vi "Pot HDI.vi"(8 "error in (no error)":errorcluster, 11 "SyringeTool Class in":refnum<class "SyringeTool Class.lvclass">) -> (0 "error out":errorcluster, 3 "SyringeTool Class out":refnum<class "SyringeTool Class.lvclass">)   [LabVIEW 2011, in "SyringeTool Class.lvclass"]
uses:
  SyringeTool Class.lvclass
  WorkTable Class/WorkTable Class.lvclass
  Vec3d Class/Vec3d Class.lvclass
panel:
  in  "Slot":u32
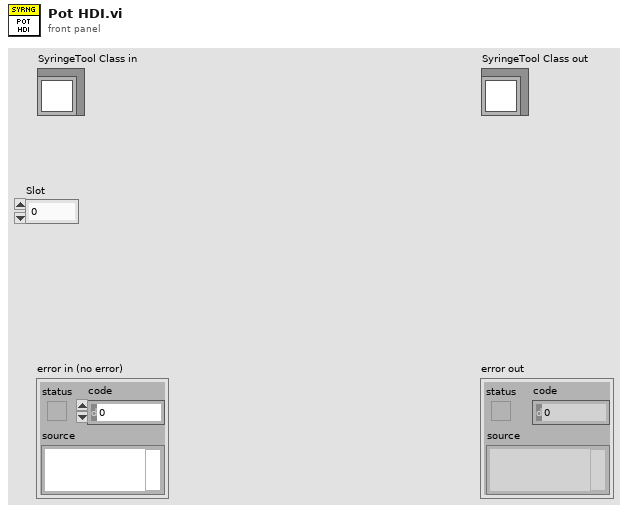
[diagram p1: front panel]
types:
  T1 = typedef "Worktable_HDI Slot.ctl" = cluster{"HDI Assembly State":enum16{"Empty", "Populated"}, "HDI Type":enum16{"HDI", "Polyimide"}, "Vacuum Channel":u32, "Location/Orientation":T2}
  T2 = typedef "Position_Orientation.ctl" = cluster{"Center":refnum<class "Vec3d Class.lvclass">, "Orientation":refnum<class "Orient3d Class.lvclass">}
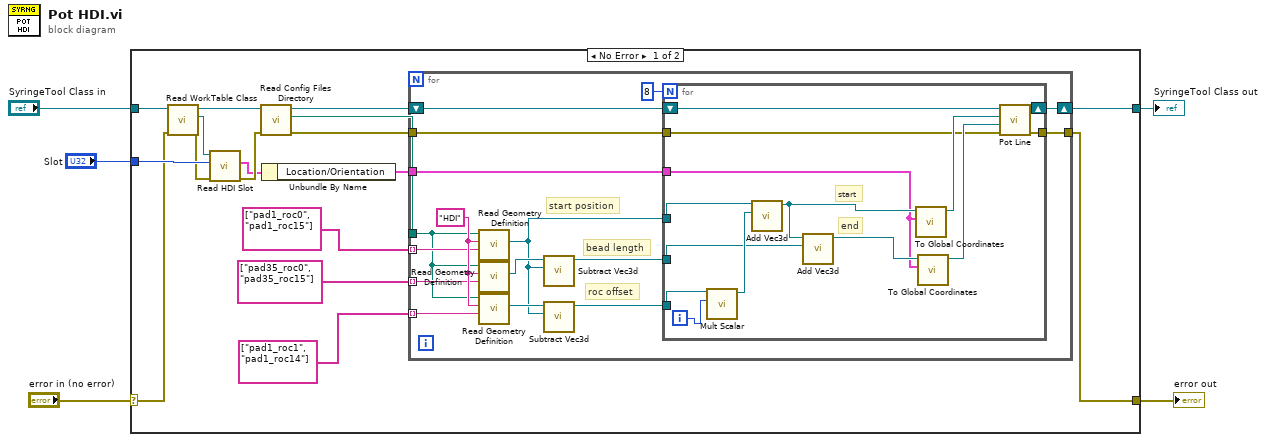
[diagram p0: block diagram]
diagram:
  n1 = case shown="No Error" "error in (no error)" {
    selector: "error in (no error)" -> [w8 w54]
    tunnel: [w6 w54] -> w4
    tunnel: [w14 w53] -> w2
    tunnel: "SyringeTool Class in" -> [w22 w53]
    tunnel: "Slot" -> [w20 _]
    frame No Error {
      n2 = call-dynamic "Read WorkTable Class.vi"("error in"=w8, "Gantry Class in"=w22) -> ("error out"=w19:errorcluster, "WorkTable Class.lvclass"=w21:refnum<class "WorkTable Class.lvclass">, "Gantry Class out"=w18:refnum<class "SyringeTool Class.lvclass">)  [unwired: 7 in]
      n3 = call-dynamic "Read HDI Slot.vi"("error in"=w19, "HDI Slot Number"=w20, "WorkTable in"=w21) -> ("error out"=w17:errorcluster, "HDI Slot"=w16:T1)  [unwired: 6 in, 1 out]
      n4 = call-dynamic "Read Config Files Directory.vi"("error in (no error)"=w17, "Gantry Class in"=w18) -> ("error out"=w7:errorcluster, "Config Files Directory"=w12:path, "Gantry Class out"=w15:refnum<class "SyringeTool Class.lvclass">)  [unwired: 7 in]
      n5 = Unbundle By Name(w16) -> ("Location/Orientation"=w9:T2)
      n6 = for {
        shift-right: [w37] -> w14
        shift-left: w15 -> [w38]
        tunnel: string[] ["pad35_roc0", "pad35_roc15"] -> [w33] mode=indexing
        tunnel: w12 -> [w30]
        tunnel: string[] ["pad1_roc0", "pad1_roc15"] -> [w32] mode=indexing
        tunnel: string[] ["pad1_roc1", "pad1_roc14"] -> [w31] mode=indexing
        tunnel: w9 -> [w26]
        tunnel: w7 -> [w24]
        tunnel: [w23] -> w6
        w36 = "HDI" ("Part")
        # "roc offset"
        # "start position"
        # "bead length"
        n7 = call "Read Geometry Definition.vi"("Feature"=w32, "Part"=w36, "Config Location"=w30) -> ("Feature Coordinates"=w29:refnum<class "Vec3d Class.lvclass">)  [unwired: 7 in, 1 out]
        n8 = call "Read Geometry Definition.vi"("Feature"=w33, "Part"=w36, "Config Location"=w30) -> ("Feature Coordinates"=w35:refnum<class "Vec3d Class.lvclass">)  [unwired: 7 in, 1 out]
        n9 = call "Read Geometry Definition.vi"("Feature"=w31, "Part"=w36, "Config Location"=w30) -> ("Feature Coordinates"=w34:refnum<class "Vec3d Class.lvclass">)  [unwired: 7 in, 1 out]
        n10 = call "Subtract Vec3d.vi"("Vec3d in 2"=w29, "Vec3d in 1"=w35) -> ("Vec3d Class out"=w28:refnum<class "Vec3d Class.lvclass">)  [unwired: 8 in, 1 out]
        n11 = call "Subtract Vec3d.vi"("Vec3d in 2"=w29, "Vec3d in 1"=w34) -> ("Vec3d Class out"=w27:refnum<class "Vec3d Class.lvclass">)  [unwired: 8 in, 1 out]
        n12 = for {
          N: 8 -> [_]
          shift-right: [w51] -> w37
          shift-left: w38 -> [w52]
          tunnel: w29 -> [w44]
          tunnel: w28 -> [w45]
          tunnel: w27 -> [w46]
          tunnel: w26 -> [w41]
          tunnel: w24 -> [w40]
          tunnel: [w39] -> w23
          i -> [w47]
          # "end"
          # "start"
          n13 = call-dynamic "Mult Scalar.vi"("Scale"=w47, "Vec3d in"=w46) -> ("Vec3d out"=w50:refnum<class "Vec3d Class.lvclass">)  [unwired: 8 in, 1 out]
          n14 = call-dynamic "Add Vec3d.vi"(10:"Vec3d Class in"=w50, 11:"Vec3d Class in"=w44) -> ("Vec3d Class out"=w49:refnum<class "Vec3d Class.lvclass">)  [unwired: 8 in, 1 out]
          n15 = call-dynamic "Add Vec3d.vi"(10:"Vec3d Class in"=w45, 11:"Vec3d Class in"=w49) -> ("Vec3d Class out"=w48:refnum<class "Vec3d Class.lvclass">)  [unwired: 8 in, 1 out]
          n16 = call "To Global Coordinates.vi"("Center/Orientation"=w41, "Local Coordinates"=w49) -> ("Global Coordinates"=w42:refnum<class "Vec3d Class.lvclass">)  [unwired: 8 in, 1 out]
          n17 = call "To Global Coordinates.vi"("Center/Orientation"=w41, "Local Coordinates"=w48) -> ("Global Coordinates"=w43:refnum<class "Vec3d Class.lvclass">)  [unwired: 8 in, 1 out]
          n18 = call-dynamic "Pot Line.vi"("error in"=w40, "End Position"=w43, "Start Position"=w42, "SyringeTool in"=w52) -> ("error out"=w39:errorcluster, "SyringeTool out"=w51:refnum<class "SyringeTool Class.lvclass">)  [unwired: 6 in]
        }
      }
    }
    frame Error {
    }
  }
  "error out" <- w4
  "SyringeTool Class out" <- w2
